vi "TimeTriggerToReport.vi"(9 "延遲(分)":i32, 10 "時間(點, 區間)":i32[][](array[numeric]), 11 "Current Time":timestamp) -> (0 "目標資料夾":string, 1 "[生成]時間點":timestamp, 2 "時間區間(End)":timestamp, 3 "時間區間(Start)":timestamp)   [LabVIEW 2019]
panel:
  out "當前時間前五分鐘":timestamp
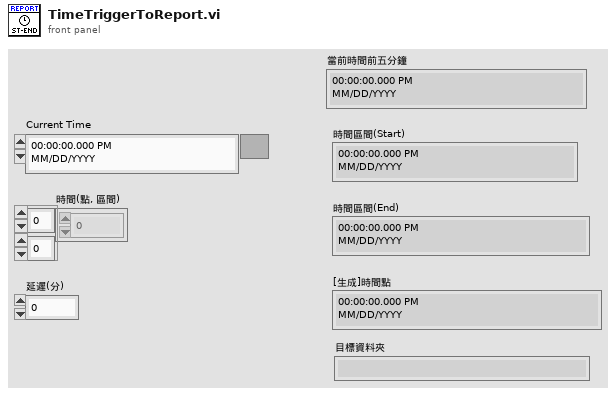
[diagram p1: front panel]
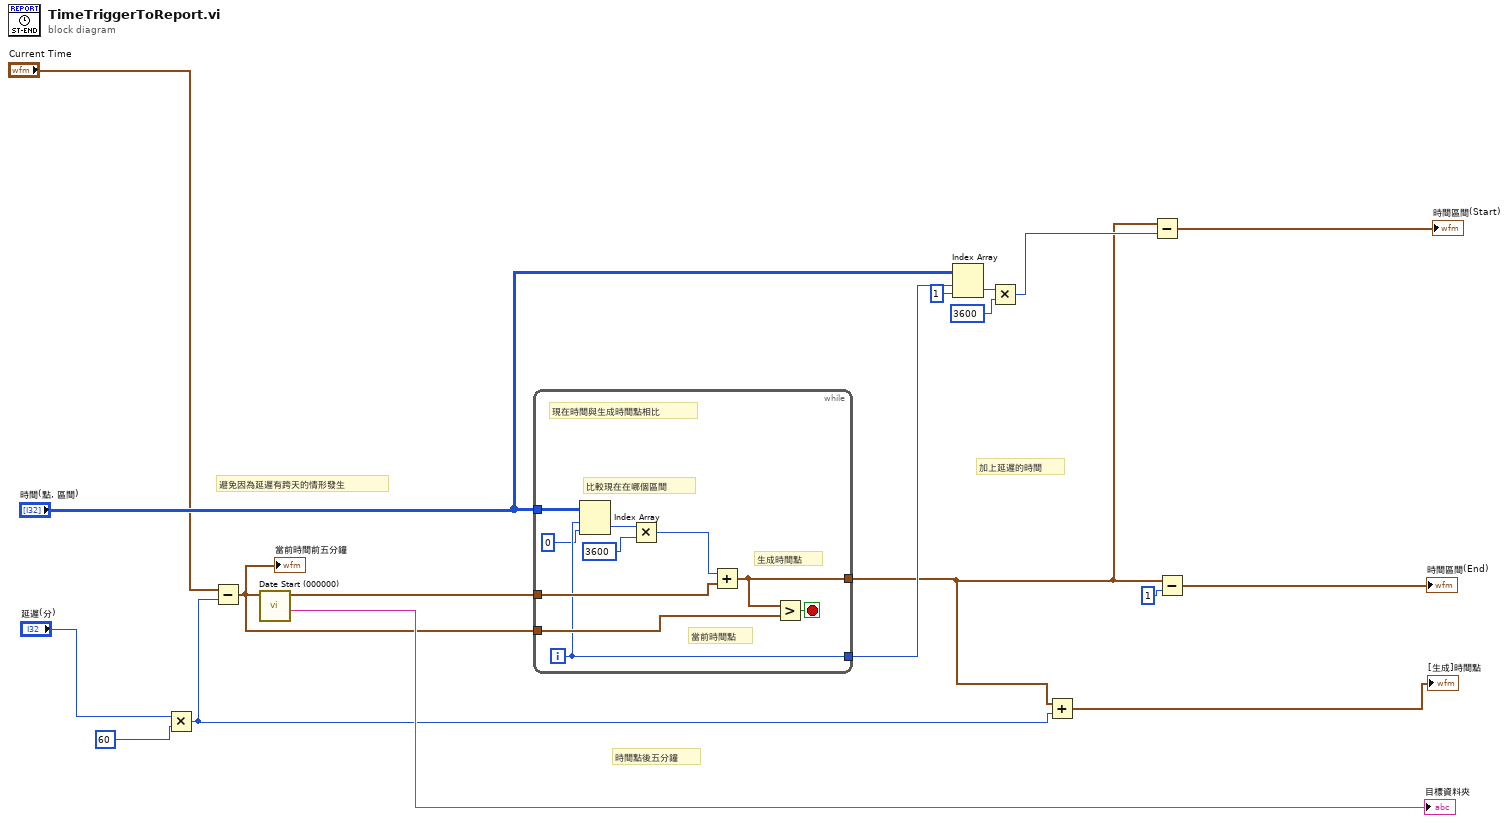
[diagram p0: block diagram]
diagram:
  # "避免因為延遲有跨天的情形發生"
  # "加上延遲的時間"
  # "時間點後五分鐘"
  n1 = Multiply(x="延遲(分)", y=60) -> (x*y=w3:i32)
  n2 = Subtract(x="Current Time", y=w3) -> (x-y=w4:timestamp)
  "當前時間前五分鐘" <- w4
  n3 = call "Date Start (000000).vi"("Datetime"=w4) -> ("檔名"=→"目標資料夾":string, "Date + 00:00:00"=w7:timestamp)  [unwired: 9 in]
  n4 = while {
    tunnel: "時間(點, 區間)" -> [w24]
    tunnel: w7 -> [w27]
    tunnel: w4 -> [w26]
    tunnel: [w25] -> w2
    tunnel: [w23] -> w11
    i -> [w23]
    stop <- w20 stop-if-true
    # "當前時間點"
    # "生成時間點"
    # "現在時間與生成時間點相比"
    # "比較現在在哪個區間"
    n5 = Index Array(array=w24, index (row)=w23, index (col)=0 ("disabled index (col)")) -> (element=w21:i32)
    n6 = Multiply(x=w21, y=3600) -> (x*y=w19:i32)
    n7 = Add(x=w19, y=w27) -> (x+y=w25:timestamp)
    n8 = Greater?(x=w25, y=w26) -> (0:w20:bool)
  }
  n9 = Index Array(array="時間(點, 區間)", index (row)=w11, index (col)=1 ("disabled index (col)")) -> (element=w13:i32)
  n10 = Multiply(x=w13, y=3600) -> (x*y=w16:i32)
  n11 = Add(x=w2, y=w3) -> (x+y=→"[生成]時間點":timestamp)
  n12 = Subtract(x=w2, y=w16) -> (x-y=→"時間區間(Start)":timestamp)
  n13 = Subtract(x=w2, y=1) -> (x-y=→"時間區間(End)":timestamp)
